vi "WaveformChart - Colors.vi"(8 "error in (no error)":errorcluster, 10 "Ctl Refnum":refnum<vi>, 11 "Material-Scheme in":refnum<class "Material-Scheme.lvclass">) -> (0 "error out":errorcluster)   [LabVIEW 2021, in "TSC Material Theme.lvlib" / "Material-Scheme.lvclass"]
doc: "Sets the colors of the waveform chart.\n\n<b>Code Developed By:</b>\nTechnology Service Corporation\n1983 S Liberty Drive\nBloomington, IN 47403\nwww.tsc.com/atcs\n\nDeveloper:\nDaniel Coons"
uses:
  Material-Scheme.lvclass
  Material-Scheme.lvclass/Material-Scheme.ctl
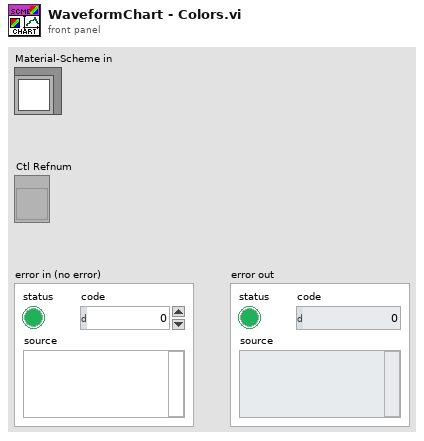
[diagram p1: front panel]
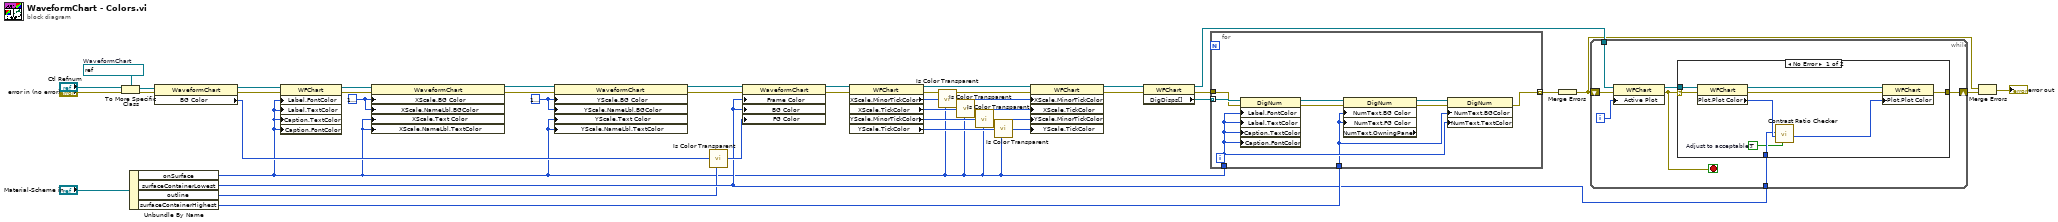
[diagram p0: block diagram]
diagram:
  w25 = u32 16777216 ("X Scale.Name Label.Colors:FG Color")
  w22 = u32 16777216 ("X Scale.Name Label.Colors:FG Color")
  w39 = refnum<vi> refnum  # WaveformChart
  n1 = To More Specific Class(target class=w39, reference="Ctl Refnum", error in="error in (no error)") -> (specific class reference=w40:refnum<vi>, error out=w41:errorcluster)
  n2 = Unbundle By Name("Material-Scheme in") -> ("onSurface"=w1:u32, "surfaceContainerLowest"=w6:u32, "outline"=w4:u32, "surfaceContainerHighest"=w33:u32)
  n3 = property class="WaveformChart"(reference=w40, error in=w41) -> (reference out=w43:refnum<vi>, error out=w42:errorcluster, "BG Color"=w5:u32)
  n4 = property class="WFChart"(reference=w43, error in=w42, "Label.FontColor"=w1, "Label.TextColor"=w1, "Caption.TextColor"=w1, "Caption.FontColor"=w1) -> (reference out=w8:refnum<vi>, error out=w7:errorcluster)
  n5 = property class="WaveformChart"(reference=w8, error in=w7, "XScale.BG Color"=w22, "XScale.NameLbl.BGColor"=w22, "XScale.Text Color"=w1, "XScale.NameLbl.TextColor"=w1) -> (reference out=w24:refnum<vi>, error out=w23:errorcluster)
  n6 = property class="WaveformChart"(reference=w24, error in=w23, "YScale.BG Color"=w25, "YScale.NameLbl.BGColor"=w25, "YScale.Text Color"=w1, "YScale.NameLbl.TextColor"=w1) -> (reference out=w27:refnum<vi>, error out=w26:errorcluster)
  n7 = call "Is Color Transparent.vi"("original color"=w5, "desired color"=w4) -> ("updated color"=w21:u32)  [unwired: 3 in]
  n8 = property class="WaveformChart"(reference=w27, error in=w26, "Frame Color"=w6, "BG Color"=w6, "FG Color"=w21) -> (reference out=w20:refnum<vi>, error out=w19:errorcluster)
  n9 = property class="WFChart"(reference=w20, error in=w19) -> (reference out=w10:refnum<vi>, error out=w9:errorcluster, "XScale.MinorTickColor"=w18:u32, "XScale.TickColor"=w16:u32, "YScale.MinorTickColor"=w14:u32, "YScale.TickColor"=w12:u32)
  n10 = call "Is Color Transparent.vi"("original color"=w18, "desired color"=w1) -> ("updated color"=w17:u32)  [unwired: 3 in]
  n11 = call "Is Color Transparent.vi"("original color"=w16, "desired color"=w1) -> ("updated color"=w15:u32)  [unwired: 3 in]
  n12 = call "Is Color Transparent.vi"("original color"=w14, "desired color"=w1) -> ("updated color"=w13:u32)  [unwired: 3 in]
  n13 = call "Is Color Transparent.vi"("original color"=w12, "desired color"=w1) -> ("updated color"=w11:u32)  [unwired: 3 in]
  n14 = property class="WFChart"(reference=w10, error in=w9, "XScale.MinorTickColor"=w17, "XScale.TickColor"=w15, "YScale.MinorTickColor"=w13, "YScale.TickColor"=w11) -> (reference out=w2:refnum<vi>, error out=w3:errorcluster)
  n15 = property class="WFChart"(reference=w2, error in=w3) -> (reference out=w30:refnum<vi>, error out=w32:errorcluster, "DigDisps[]"=w35:refnum<vi>[])
  n16 = for {
    tunnel: w35 -> [w48] mode=indexing
    tunnel: [w47] -> w34 mode=indexing
    tunnel: w1 -> [w46]
    tunnel: w33 -> [w45]
    tunnel: w32 -> [w44]
    n17 = property class="DigNum"(reference=w48, error in=w44, "Label.FontColor"=w46, "Label.TextColor"=w46, "Caption.TextColor"=w46, "Caption.FontColor"=w46) -> (reference out=w51:refnum<vi>, error out=w49:errorcluster)
    n18 = property class="DigNum" props=["NumText", "BG Color", "NumText", "FG Color", "NumText", "OwningPane"](reference=w51, error in=w49, "NumText.BG Color"=w45, "NumText.FG Color"=w45) -> (reference out=w52:refnum<vi>, error out=w50:errorcluster)  [unwired: 1 out]
    n19 = property class="DigNum"(reference=w52, error in=w50, "NumText.BGColor"=w45, "NumText.TextColor"=w46) -> (error out=w47:errorcluster)  [unwired: 1 out]
  }
  n20 = Merge Errors(w34) -> (w28:errorcluster)
  n21 = while {
    tunnel: w30 -> [w58]
    shift-right: [w55] -> w31
    shift-left: w28 -> [w59]
    tunnel: w6 -> [w53]
    i -> [w57]
    stop <- w56 stop-if-true
    n22 = property class="WFChart"(reference=w58, error in=w59, "Active Plot"=w57) -> (reference out=w54:refnum<vi>, error out=w56:errorcluster)
    n23 = case shown="No Error" w56 {
      selector: w56 -> [w68 _]
      tunnel: [w62 _] -> w55
      tunnel: w54 -> [w67 _]
      tunnel: w53 -> [w65 _]
      frame No Error {
        w64 = TRUE  # Adjust to acceptable?
        n24 = property class="WFChart"(reference=w67, error in=w68) -> (reference out=w61:refnum<vi>, error out=w63:errorcluster, "Plot.Plot Color"=w66:u32)
        n25 = call "Contrast Ratio Checker.vi"("Adjust to acceptable?"=w64, "On Color"=w66, "Background Color"=w65) -> ("Adjusted Color"=w60:u32)  [unwired: 6 in, 2 out]
        n26 = property class="WFChart"(reference=w61, error in=w63, "Plot.Plot Color"=w60) -> (error out=w62:errorcluster)  [unwired: 1 out]
      }
      frame Error {
      }
    }
  }
  n27 = Merge Errors(w28, w31) -> (→"error out":errorcluster)
